vi "ATS_SetTrigger_4Ch.vi"(6 "EngineY (K)":enum16{"J", "K"}(ring)=enum."K", 7 "EngineX (J)":enum16{"J", "K"}(ring), 8 "Engine Y":T1={"Source"=enum."Disable", "Slope"=enum."Positive", "Level"=128}, 9 "Engine X":T1={"Source"=enum."Chan_A", "Slope"=enum."Positive", "Level"=128}, 10 "TrigOperation":T3, 11 "DeviceIn":i32) -> (0 "Return Code":u32, 3 "DeviceOut":i32)   [LabVIEW 2015]
doc: "_____AlazarTech, Scope_____\n\nConfigure the trigger circuitry."
uses:
  ATS_ctl/ATS_TriggerEngine_4Ch.ctl
  ATS_ctl/ATS_TriggerSource_4Ch.ctl
  ATS_ctl/TriggerOperation.ctl
  ATS_ctl/ATS_Global_Ctrl.ctl
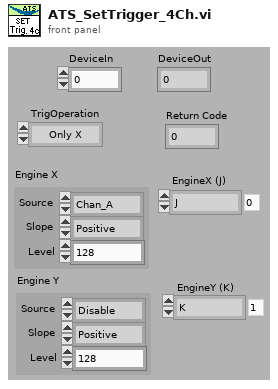
[diagram p1: front panel]
types:
  T1 = typedef "ATS_TriggerEngine_4Ch.ctl" = cluster{"Source":T2, "Slope":enum32{"Positive", "Negative"}, "Level":u32}
  T2 = typedef "ATS_TriggerSource_4Ch.ctl" = enum32{"Chan_A", "Chan_B", "External", "Disable", "Chan_C", "Chan_D"}
  T3 = typedef "TriggerOperation.ctl" = enum16{"Only X", "Only Y", "X or Y", "X and Y", "X xor Y", "X and not Y", "not X and Y"}
  T4 = typedef "ATS_Global_Ctrl.ctl" = enum16{"Init_Device", "Clear_ALL", "Set", "Get"}
  T5 = typedef "ATS_Set_Value.ctl" = cluster{"Clock (s)":dbl, "RangeA (v)":dbl, "RangeB (v)":dbl, "Ranges (v)":dbl[]}
  T6 = typedef "ATS_Global_4Ch.ctl" = cluster{"Record":T7, "Clock":T8, "Inputs":T12, "Trigger":T18}
  T7 = typedef "Record.ctl" = cluster{"Count":u32, "Presize":u32, "Length":u32}
  T8 = typedef "Clock.ctl" = cluster{"ClckSource":T9, "ClckRate":T10, "ClckEdge":T11, "Decimation":u32}
  T9 = typedef "ClockSource.ctl" = enum16{"Internal", "External", "Medium Ext.", "Slow Ext.", "Ext. AC", "Ext. DC", "Ext. (PLL)"}
  T10 = typedef "ClockRate.ctl" = u32
  T11 = typedef "ClockEdge.ctl" = u16
  T12 = typedef "ATS_InputArray.ctl" = T13[]
  T13 = typedef "InputCtrl.ctl" = cluster{"Coupling":T14, "Range":T15, "Impedance":T16, "Bandwidth":T17}
  T14 = typedef "Coupling.ctl" = enum16{"AC", "DC"}
  T15 = typedef "Range.ctl" = u32
  T16 = typedef "Impedance.ctl" = enum16{"1M ohms", "50 ohms"}
  T17 = typedef "Bandwidth.ctl" = enum16{"Full Bandwidth", "Reduce Bandwidth"}
  T18 = typedef "ATS_Trigger_4Ch.ctl" = cluster{"TrigOperation":T3, "Timeout (s)":dbl, "Trig. Delay":u32, "Engine X":T1, "Engine Y":T1, "ExtTrigControl":T19}
  T19 = typedef "ExtTrigger.ctl" = cluster{"Coupling":T14, "Range":T20}
  T20 = typedef "ExtTrigRange.ctl" = enum16{"1 V", "5 V", "TTL"}
  T21 = typedef "Device_Info.ctl" = cluster{"Handle":u32, "Board":string, "CPLD":string, "MemorySize":u32, "SampleSize":u8, "ID":i32, "High_Memory":bool, "Chan/Board":u8}
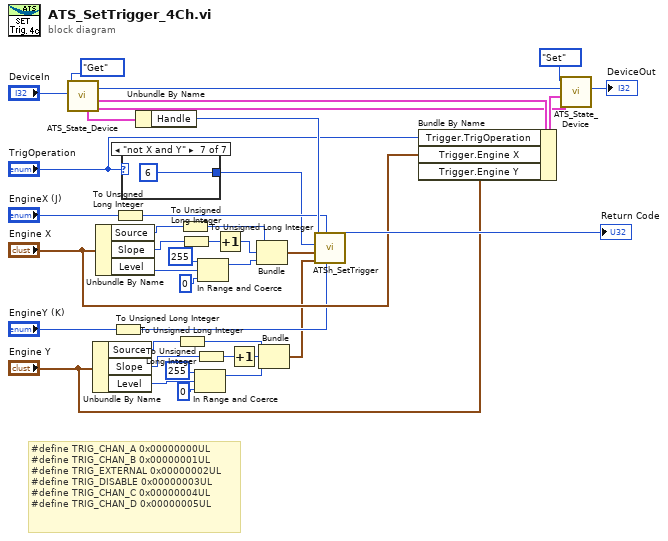
[diagram p0: block diagram]
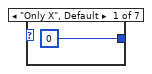
[diagram p2: hidden frame]
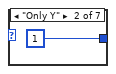
[diagram p3: hidden frame]
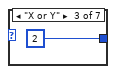
[diagram p4: hidden frame]
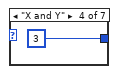
[diagram p5: hidden frame]
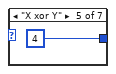
[diagram p6: hidden frame]
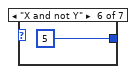
[diagram p7: hidden frame]
diagram:
  # "#define TRIG_CHAN_A 0x00000000UL\n#define TRIG_CHAN_B 0x00000001UL\n#define TRIG_EXTERNAL 0x00000002UL\n#define TRIG_DISABLE 0x00000003UL\n#define TRIG_CHAN_C 0x00000004UL\n#define TRIG_CHAN_D 0x00000005UL"
  n1 = call "ATS_State_Device.vi"("DeviceIn"="DeviceIn", "ATS_GBL_Ctrl"=ATS_Global_Ctrl."Get") -> ("Ref_Out"=w12:T5, "SetupOut"=w14:T6, "DeviceOut"=w22:i32, "DevInfo_Out"=w13:T21)  [unwired: 4 in, 2 out]
  n2 = Unbundle By Name("Engine Y") -> ("Source"=w27:T2, "Slope"=w28:enum32{"Positive", "Negative"}, "Level"=w29:u32)
  n3 = Unbundle By Name("Engine X") -> ("Source"=w37:T2, "Slope"=w36:enum32{"Positive", "Negative"}, "Level"=w35:u32)
  n4 = To Unsigned Long Integer(number="EngineY (K)") -> (unsigned 32bit integer=w11:u32)
  n5 = To Unsigned Long Integer(number="EngineX (J)") -> (unsigned 32bit integer=w10:u32)
  n6 = case shown="\"not X and Y\"" "TrigOperation" {
    tunnel: [u32 0 ("Operation") u32 1 ("Operation") u32 2 ("Operation") u32 3 ("Operation") u32 4 ("Operation") u32 5 ("Operation") u32 6 ("Operation")] -> w9
    frame "Only X", Default {
    }
    frame "Only Y" {
    }
    frame "X or Y" {
    }
    frame "X and Y" {
    }
    frame "X xor Y" {
    }
    frame "X and not Y" {
    }
    frame "not X and Y" {
    }
  }
  n7 = Unbundle By Name(w13) -> ("Handle"=w18:u32)
  n8 = To Unsigned Long Integer(number=w27) -> (unsigned 32bit integer=w4:u32)
  n9 = To Unsigned Long Integer(number=w37) -> (unsigned 32bit integer=w7:u32)
  n10 = To Unsigned Long Integer(number=w36) -> (unsigned 32bit integer=w34:u32)
  n11 = In Range and Coerce(upper limit=u32 255, x=w29, lower limit=u32 0) -> (coerced(x)=w3:u32)  [unwired: 1 out]
  n12 = To Unsigned Long Integer(number=w28) -> (unsigned 32bit integer=w25:u32)
  n13 = In Range and Coerce(upper limit=u32 255, x=w35, lower limit=u32 0) -> (coerced(x)=w5:u32)  [unwired: 1 out]
  n14 = Increment(x=w34) -> (x+1=w6:u32)
  n15 = Increment(x=w25) -> (x+1=w2:u32)
  n16 = Bundle(w7, w6, "upper limit"=w5) -> (w8:cluster{u32, u32, "upper limit":u32})  [unwired: 1 in]
  n17 = Bundle(w4, w2, "upper limit"=w3) -> (w1:cluster{u32, u32, "upper limit":u32})  [unwired: 1 in]
  n18 = call "ATSh_SetTrigger.vi"("EngineY(1)"=w11, "EngineX(0)"=w10, "EngineY"=w1, "EngineX"=w8, "Operation"=w9, "Handle"=w18) -> ("Return"=→"Return Code":u32)  [unwired: 4 in, 1 out]
  n19 = Bundle By Name(cluster=w14, "Trigger.TrigOperation"="TrigOperation", "Trigger.Engine X"="Engine X", "Trigger.Engine Y"="Engine Y") -> (w19:T6)
  n20 = call "ATS_State_Device.vi"("Ref_In"=w12, "SetupIn"=w19, "DeviceIn"=w22, "ATS_GBL_Ctrl"=ATS_Global_Ctrl."Set") -> ("DeviceOut"=→"DeviceOut":i32)  [unwired: 2 in, 5 out]
